vi "Get State.vi"(8 "error in (no error)":errorcluster, 11 "Command Processor Actor in":refnum<class "Command Processor Actor.lvclass">) -> (0 "error out":errorcluster, 1 "State String":string, 3 "Command Processor Actor out":refnum<class "Command Processor Actor.lvclass">)   [LabVIEW 2014, in "Robot Actor Framework.lvlib" / "Command Processor Actor.lvlib" / "Command Processor Actor.lvclass"]
uses:
  Command Processor Actor.lvclass
  Command Processor Actor.lvclass/Command Processor Actor.ctl
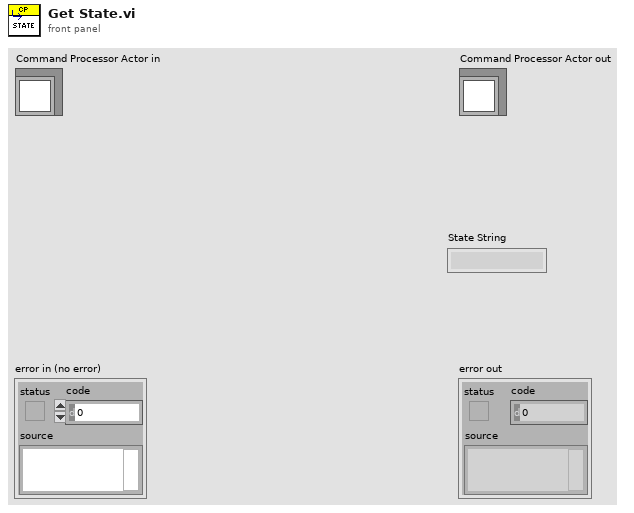
[diagram p1: front panel]
types:
  T1 = typedef "Robot Actor Framework.lvlib/Command Processor Actor.lvlib/Command Processor Actor.lvclass/Command Processor States.ctl" = enum16{"Unknown", "No Command", "Running Command", "Starting Command", "Stopping Command", "Finishing Command"}
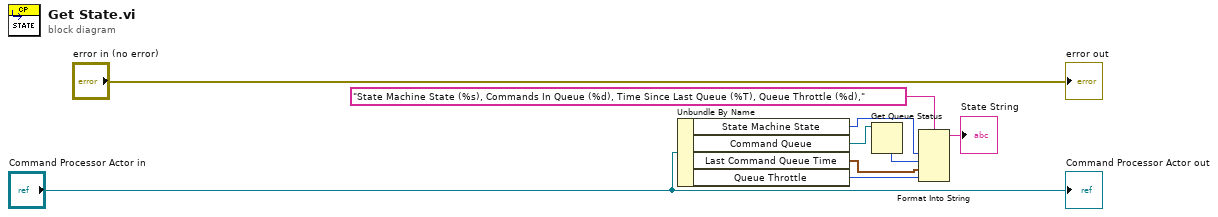
[diagram p0: block diagram]
diagram:
  n1 = Unbundle By Name("Command Processor Actor in") -> ("State Machine State"=w5:T1, "Command Queue"=w7:refnum<queue>, "Last Command Queue Time"=w3:timestamp, "Queue Throttle"=w2:u32)
  n2 = Get Queue Status(queue=w7) -> (# elements in queue=w4:i32)  [unwired: 2 in, 7 out]
  n3 = Format Into String(format string="State Machine State (%s), Commands In Queue (%d), Time Since Last Queue (%T), Queue Throttle (%d),", w5, w4, w3, w2) -> (resulting string=→"State String":string)  [unwired: 2 in, 1 out]
  "error out" <- "error in (no error)"
  "Command Processor Actor out" <- "Command Processor Actor in"
